vi "LDA Save.vi"(8 "error in":errorcluster, 10 "File Path":path, 11 "LDA":refnum<class "LDA.lvclass">) -> (0 "error out":errorcluster, 3 "LDA":refnum<class "LDA.lvclass">)   [LabVIEW 2020, in "OpenLvVision_OpenCv.lvlib" / "LDA.lvclass"]
doc: "Serializes this object."
uses:
  LDA.lvclass
  C:/Users/lukas/Downloads/OpenLvVision_OpenCv/SourceCode/LabView/OpenLvVision_OpenCv/_LvHelpers/EdvrObject/EdvrObject.lvclass
  _LvHelpers/EdvrObject/EdvrObject.lvclass/EdvrObject.ctl
  OpenLvVision_OpenCv.lvlib
  _LvHelpers/EdvrObject/EdvrObject.lvclass
  Dlls/OlvOpenCvWrapper.dll
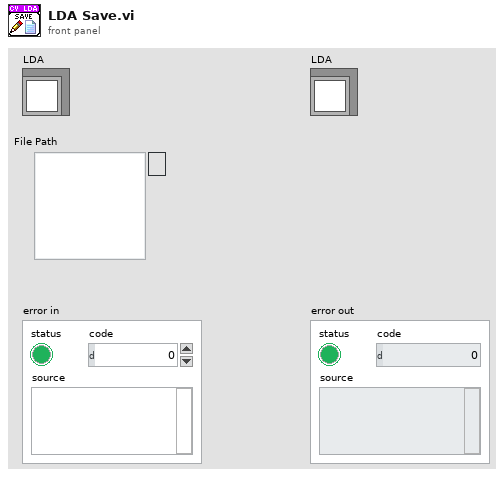
[diagram p1: front panel]
types:
  T1 = typedef "OpenLvVision_OpenCv.lvlib/EdvrObject.lvclass/Edvr.ctl" = refnum<data-value>
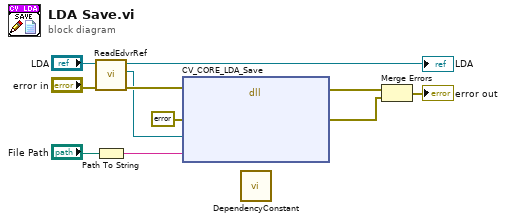
[diagram p0: block diagram]
diagram:
  n1 = call "ReadEdvrRef.vi"("error in (no error)"="error in", "EdvrObject in"="LDA") -> ("error out"=w4:errorcluster, "Edvr"=w3:T1, "EdvrObject out"=→"LDA":refnum<class "LDA.lvclass">)  [unwired: 7 in]
  n2 = Path To String(path="File Path") -> (string=w1:string)
  n3 = dll-call lib="C:/Users/lukas/Downloads/OpenLvVision_OpenCv/SourceCode/LabView/OpenLvVision_OpenCv/Dlls/OlvOpenCvWrapper.dll" fn="CV_CORE_LDA_Save"(error in=w4, "Error"=errorcluster {"status"=FALSE, "code"=0, "source"=""} ("error out"), "edvrRef"=w3, "filePath"=w1) -> (error out=w6:errorcluster, "Error"=w5:errorcluster)  [unwired: 5 in, 1 out]
  n4 = call "DependencyConstant.vi"() -> ()  [unwired: 12 in]
  n5 = Merge Errors(w6, w5) -> (→"error out":errorcluster)
